vi "LV2 Global.vi"(10 "Write":bool, 11 "Boolean In":bool) -> (3 "Boolean":bool)   [LabVIEW 2021]
panel:
  in  "Index":i32
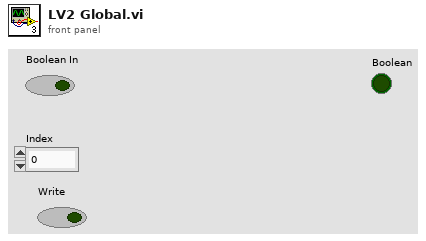
[diagram p1: front panel]
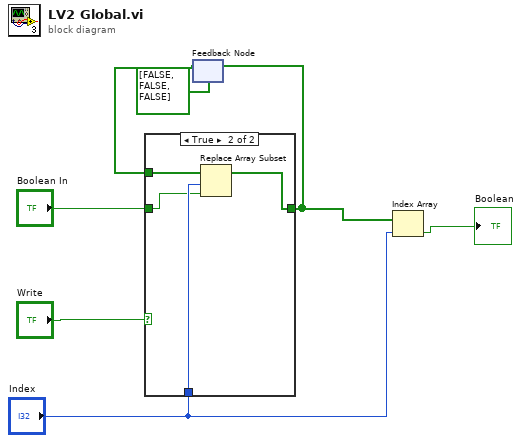
[diagram p0: block diagram]
diagram:
  n1 = feedback #1(bool[] [FALSE, FALSE, FALSE] ("Boolean In")) -> (w5:bool[])
  n2 = case shown="True" "Write" {
    tunnel: "Boolean In" -> [_ w9]
    tunnel: [w8 w11] -> w3
    tunnel: w5 -> [w8 w12]
    tunnel: "Index" -> [_ w10]
    frame False {
    }
    frame True {
      n3 = Replace Array Subset(array=w12, new element=w9, index=w10) -> (w11:bool[])
    }
  }
  n4 = feedback-in #1(w3) -> ()
  n5 = Index Array(array=w3, index="Index") -> (element=→"Boolean":bool)
